vi "get_magnification.vi"(8 "error in (no error)":errorcluster, 11 "GenericObjective in":refnum<class "GenericObjective.lvclass">) -> (0 "error out":errorcluster, 1 "calibrated magnification":dbl, 2 "magnification":dbl=1.0, 3 "GenericObjective out":refnum<class "GenericObjective.lvclass">, 4 "nominal magnification":i32)   [LabVIEW 2010, in "GenericObjective.lvclass"]
uses:
  GenericObjective.lvclass
  GenericObjective.lvclass/GenericObjective.ctl
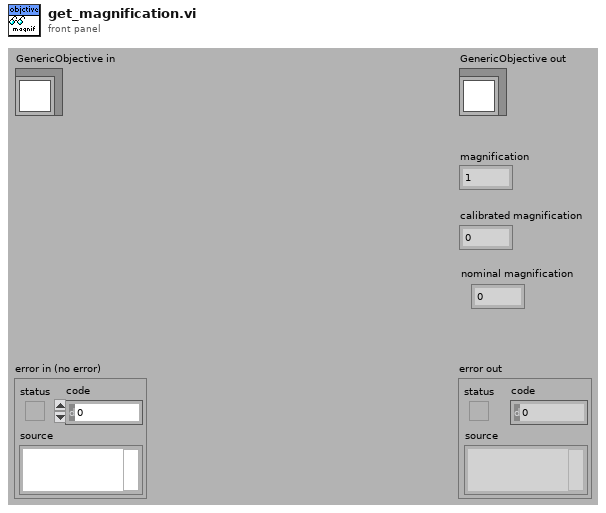
[diagram p1: front panel]
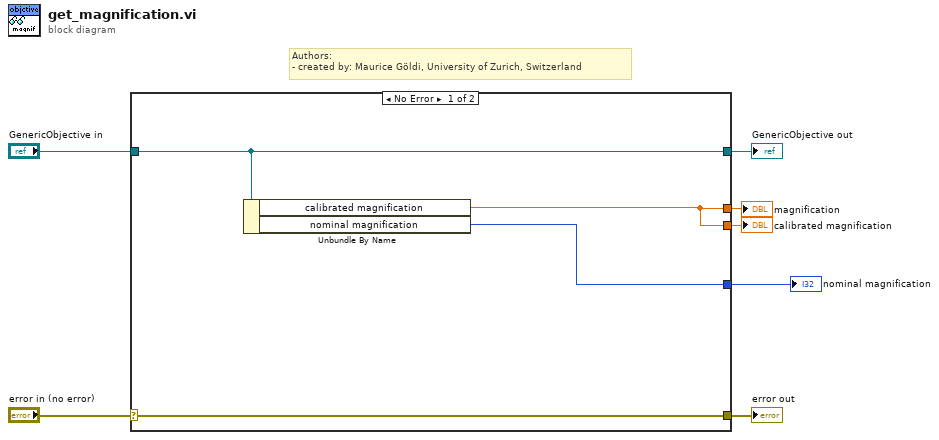
[diagram p0: block diagram]
diagram:
  # "Authors: \n- created by: Maurice Göldi, University of Zurich, Switzerland"
  n1 = case shown="No Error" "error in (no error)" {
    selector: "error in (no error)" -> [w11 w13]
    tunnel: [w11 w13] -> w6
    tunnel: [w10 w12] -> w4
    tunnel: "GenericObjective in" -> [w10 w12]
    tunnel: [w9 _] -> w3
    tunnel: [w9 _] -> w2
    tunnel: [w8 _] -> w1
    frame No Error {
      n2 = Unbundle By Name(w10) -> ("calibrated magnification"=w9:dbl, "nominal magnification"=w8:i32)
    }
    frame Error {
    }
  }
  "error out" <- w6
  "GenericObjective out" <- w4
  "magnification" <- w3
  "calibrated magnification" <- w2
  "nominal magnification" <- w1
